vi "Determine Features from String.vi"(8 "error in (no error)":errorcluster, 10 "Features":string, 11 "FTP in":refnum<class "FTP.lvclass">) -> (0 "error out":errorcluster, 3 "FTP out":refnum<class "FTP.lvclass">)   [LabVIEW 2013, in "FTP.lvlib" / "FTP.lvclass"]
uses:
  FTP.lvclass
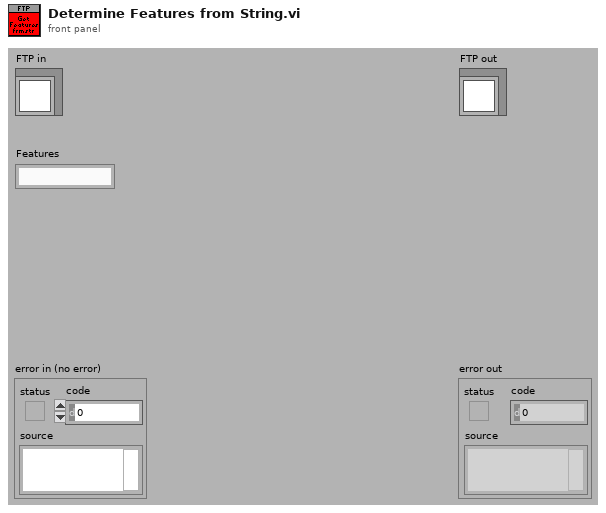
[diagram p1: front panel]
types:
  T1 = typedef "FTP.lvlib/FTP.lvclass/Features.ctl" = cluster{"SIZE":bool, "MLST":bool, "MLSD":bool, "MDTM":bool}
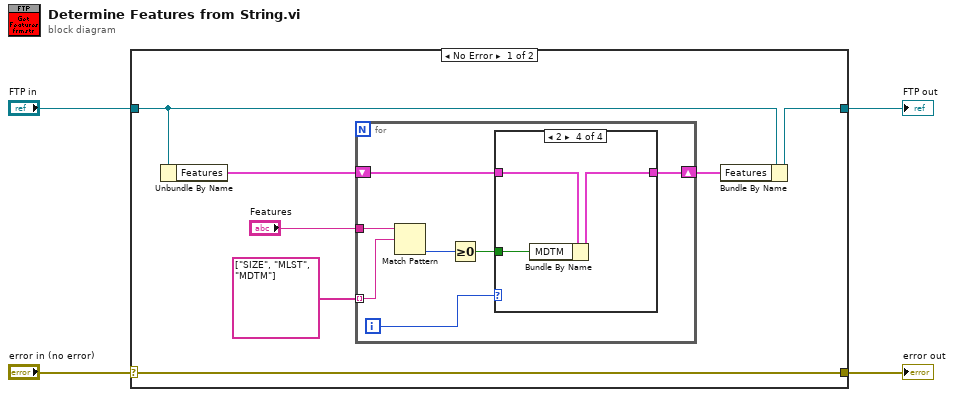
[diagram p0: block diagram]
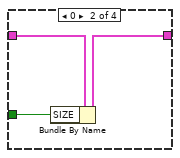
[diagram p3: hidden frame]
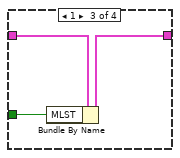
[diagram p4: hidden frame]
diagram:
  n1 = case shown="No Error" "error in (no error)" {
    selector: "error in (no error)" -> [w11 w30]
    tunnel: [w11 w30] -> w3
    tunnel: [w6 w29] -> w1
    tunnel: "FTP in" -> [w8 w29]
    frame No Error {
      n2 = Unbundle By Name(w8) -> ("Features"=w7:T1)
      n3 = for {
        tunnel: "Features" -> [w18]
        tunnel: string[] ["SIZE", "MLST", "MDTM"] -> [w17] mode=indexing
        shift-right: [w12] -> w5
        shift-left: w7 -> [w13]
        i -> [w15]
        n4 = Match Pattern(string=w18, regular expression=w17) -> (offset past match=w16:i32)  [unwired: 1 in, 3 out]
        n5 = Greater Or Equal To 0?(x=w16) -> (x >= 0?=w14:bool)
        n6 = case shown="2" w15 {
          tunnel: w14 -> [_ w21 w24 w27]
          tunnel: w13 -> [w19 w22 w25 w28]
          tunnel: [w19 w20 w23 w26] -> w12
          frame Default {
          }
          frame 0 {
            n7 = Bundle By Name(cluster=w22, "SIZE"=w21) -> (w20:T1)
          }
          frame 1 {
            n8 = Bundle By Name(cluster=w25, "MLST"=w24) -> (w23:T1)
          }
          frame 2 {
            n9 = Bundle By Name(cluster=w28, "MDTM"=w27) -> (w26:T1)
          }
        }
      }
      n10 = Bundle By Name(cluster=w8, "Features"=w5) -> (w6:refnum<class "FTP.lvclass">)
    }
    frame Error {
    }
  }
  "error out" <- w3
  "FTP out" <- w1
